vi "Actor Core.vi"(8 "error in":errorcluster, 11 "Hardware Buzzer in":refnum<class "Hardware Buzzer.lvclass">) -> (0 "error out":errorcluster, 3 "Actor out":refnum<class "Actor.lvclass">)   [LabVIEW 2023, in "Hardware Buzzer.lvlib" / "Hardware Buzzer.lvclass"]
doc: "<p>(<strong>Filename</strong>: <span class=\"dnl\">Actor Framework.lvlib:Actor.lvclass:Actor Core.vi</span>)</p>\n<p>Receives messages to the actor, reacts to them, and initiates any error handling that may shut the actor down.</p>\n<p>Descendant classes may override this VI to append parallel tasks for the actor to complete while it handles messages. Overrides use the <a href=\"nihelplauncher://docs/csh?context=lvcore_glang_udclass\">Call Parent Class Method</a> node.</p>"
uses:
  Hardware Buzzer.lvclass
  C:/Program Files/National Instruments/LabVIEW 2024/vi.lib/ActorFramework/Actor/Actor.lvclass
  <vilib>/ActorFramework/Actor/Actor.lvclass
  <vilib>/ActorFramework/Actor/Actor.lvclass/Actor.ctl
  Hardware Buzzer.lvclass/Hardware Buzzer.ctl
  <vilib>/ActorFramework/Message Enqueuer/Message Enqueuer.lvclass/Message Enqueuer.ctl
  Controller/Controller Messages/Set DAQ Panel Reference Msg/Set DAQ Panel Reference Msg.lvclass/Set DAQ Panel Reference Msg.ctl
  Controller/Controller Messages/Buzzer Pressed Msg/Buzzer Pressed Msg.lvclass/Buzzer Pressed Msg.ctl
  <vilib>/DAQmx/read.llb/DAQmx Read (Analog 1D Wfm NChan NSamp).vi
  <vilib>/ActorFramework/Message Enqueuer/Init from Existing Queue.vi
  <vilib>/ActorFramework/Message Enqueuer/Enqueue.vi
  Controller/Controller Messages/Set DAQ Panel Reference Msg/Set DAQ Panel Reference Msg.lvclass
  C:/Program Files/National Instruments/LabVIEW 2024/vi.lib/ActorFramework/Message/Message.lvclass
  Controller/Controller Messages/Buzzer Pressed Msg/Buzzer Pressed Msg.lvclass
  <vilib>/ActorFramework/Stop Msg/Stop Msg.lvclass
  <vilib>/DAQmx/create/channels.llb/DAQmx Create Channel (AI-Voltage-Basic).vi
  <vilib>/DAQmx/configure/timing.llb/DAQmx Timing (Sample Clock).vi
  <vilib>/ActorFramework/Message Priority Queue/Priority Enqueue.vi
  <vilib>/DAQmx/miscellaneous.llb/DAQmx Fill In Error Info.vi
  <vilib>/measure/mamon.llb/Trigger Detection for N Channel.vi
  <vilib>/ActorFramework/Message Enqueuer/Message Enqueuer.lvclass
  <vilib>/measure/NI_MAPro.lvlib
panel:
  out "Waveform Chart":waveform(dbl)[](graph)
  in  "Stop":bool
  in  "3":bool
  in  "2":bool
  in  "1":bool
  in  "0":bool
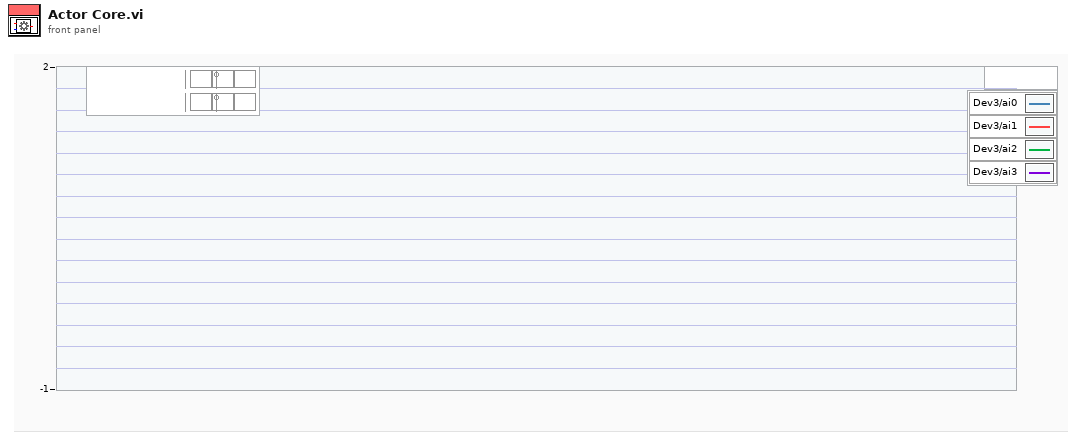
[diagram p1: front panel]
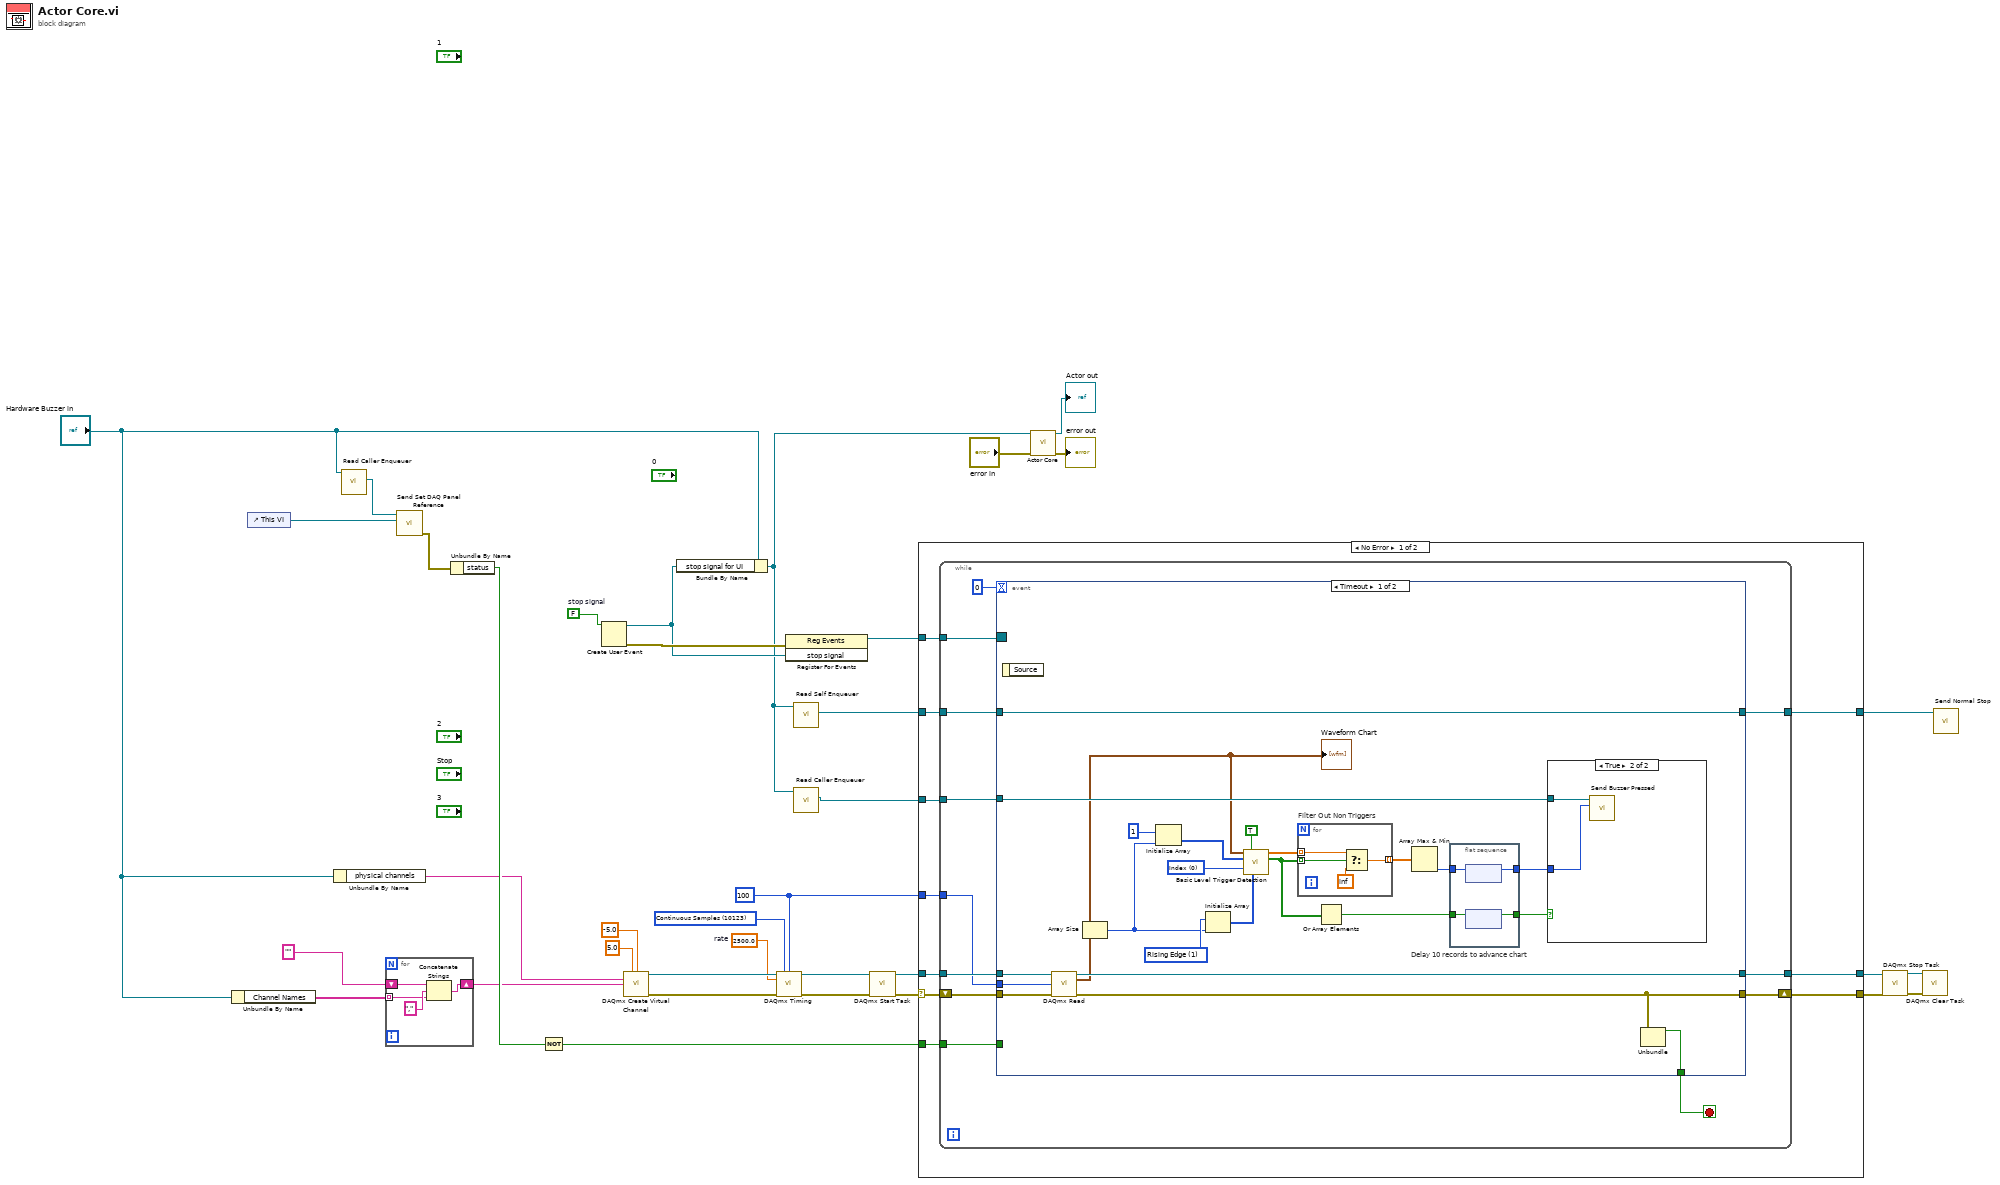
[diagram p0: block diagram]
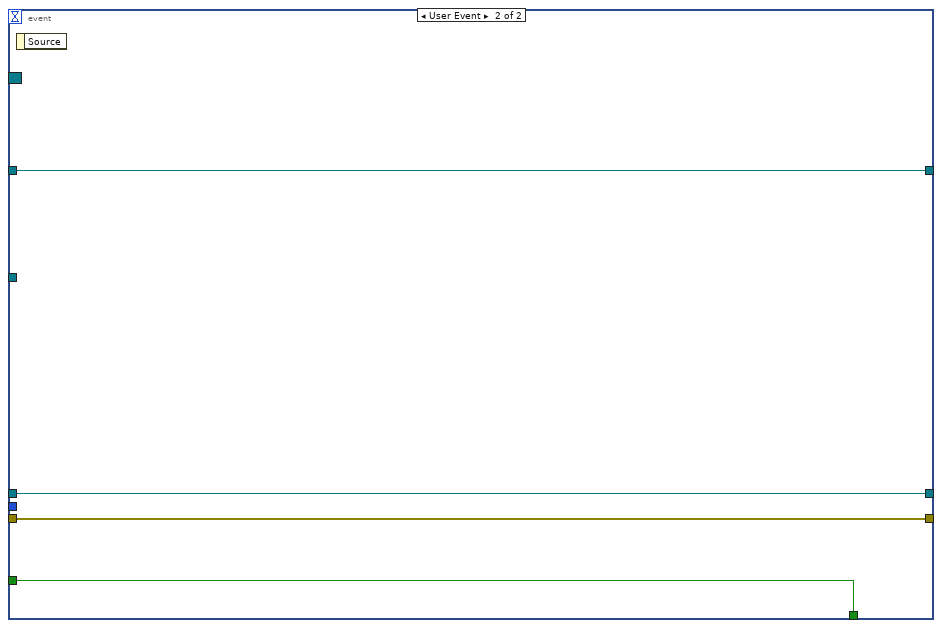
[diagram p3: hidden frame]
diagram:
  w16 = 2500.0  # rate
  w15 = 100 ("samples per channel")
  w17 = 10123 items=["Finite Samples"=10178, "Continuous Samples"=10123, "Hardware Timed Single Point"=12522] ("sample mode")
  w31 = FALSE  # stop signal
  n1 = Unbundle By Name("Hardware Buzzer in") -> ("Channel Names"=w5:string[])
  n2 = control-ref of="This VI"() -> (w29:refnum<vi>)
  n3 = Unbundle By Name("Hardware Buzzer in") -> ("physical channels"=w1:tag)
  n4 = call <vilib>:"Read Caller Enqueuer.vi"("Actor"="Hardware Buzzer in") -> ("Caller Enqueuer"=w30:refnum<class "Message Enqueuer.lvclass">)  [unwired: 10 in]
  n5 = for {
    tunnel: w5 -> [w39] mode=indexing
    shift-right: [w38] -> w4
    shift-left: "" -> [w37]
    n6 = Concatenate Strings(w37, "," ("string"), w39) -> (w38:string)
  }
  n7 = call "Send Set DAQ Panel Reference.vi"("DAQ VI Reference"=w29, "Message Enqueuer"=w30) -> ("error out"=w20:errorcluster)  [unwired: 8 in, 1 out]
  n8 = Unbundle By Name(w20) -> ("status"=w18:bool)
  n9 = Not(x=w18) -> (.not. x?=w19:bool)
  n10 = Create User Event(user event datatype=w31) -> (user event=w32:refnum<user-event>, error out=w33:errorcluster)  [unwired: 1 in]
  n11 = call-poly <vilib>:"DAQmx Create Virtual Channel.vi"("maximum value"=5.0, "minimum value"=-5.0, "physical channels"=w1, "name to assign"=w4) -> ("task out"=w28:refnum<k21>, "error out"=w13:errorcluster)  [unwired: 10 in]
  n12 = Bundle By Name(cluster="Hardware Buzzer in", "stop signal for UI"=w32) -> (w24:refnum<class "Hardware Buzzer.lvclass">)
  n13 = call-poly <vilib>:"DAQmx Timing.vi"("task/channels in"=w28, "sample mode"=w17, "samples per channel"=w15, "rate"=w16, "error in"=w13) -> ("task out"=w11:refnum<k21>, "error out"=w14:errorcluster)  [unwired: 9 in]
  n14 = register-events(error in=w33, w32) -> (reference out=w21:refnum<event-registration>)  [unwired: 1 in, 1 out]
  n15 = call <vilib>:"Read Self Enqueuer.vi"("Actor"=w24) -> ("Self Enqueuer"=w23:refnum<class "Message Enqueuer.lvclass">)  [unwired: 10 in]
  n16 = call <vilib>:"Read Caller Enqueuer.vi"("Actor"=w24) -> ("Caller Enqueuer"=w25:refnum<class "Message Enqueuer.lvclass">)  [unwired: 10 in]
  n17 = call <vilib>:"DAQmx Start Task.vi"("task/channels in"=w11, "error in"=w14) -> ("task out"=w10:refnum<k21>, "error out"=w12:errorcluster)  [unwired: 12 in]
  n18 = case shown="No Error" w12 {
    selector: w12 -> [w44 w100]
    tunnel: w25 -> [w50 _]
    tunnel: w23 -> [w49 w102]
    tunnel: [w48 w102] -> w22
    tunnel: w21 -> [w47 _]
    tunnel: w19 -> [w46 _]
    tunnel: w15 -> [w45 _]
    tunnel: w10 -> [w43 w101]
    tunnel: [w42 w100] -> w9
    tunnel: [w41 w101] -> w8
    frame No Error {
      n19 = while {
        tunnel: w43 -> [w62]
        tunnel: w50 -> [w61]
        tunnel: w49 -> [w59]
        tunnel: [w58] -> w48
        tunnel: w47 -> [w56]
        tunnel: w46 -> [w55]
        tunnel: w45 -> [w54]
        shift-right: [w52] -> w42
        shift-left: w44 -> [w53]
        tunnel: [w51] -> w41
        stop <- w57 stop-if-true
        n20 = event shown="[0] Timeout" {
          selector: w56 -> [_ _]
          dyn-events: _ -> [_ _]
          timeout: 0 -> [_ _]
          tunnel: w62 -> [w85 w96]
          tunnel: w61 -> [w84 _]
          tunnel: w59 -> [w83 w99]
          tunnel: [w83 w99] -> w58
          tunnel: [w65 w98] -> w57
          tunnel: w55 -> [_ w98]
          tunnel: w54 -> [w82 _]
          tunnel: w53 -> [w81 w97]
          tunnel: [w66 w97] -> w52
          tunnel: [w64 w96] -> w51
          event Timeout {
            w76 = u16 1 items=["Falling Edge", "Rising Edge"] ("trigger slope")
            w80 = u16 0 items=["Index", "Time"] ("location mode")
            n21 = event-data() -> ()  [unwired: 1 in, 1 out]
            n22 = call-poly <vilib>:"DAQmx Read.vi"("task/channels in"=w85, "number of samples per channel"=w82, "error in"=w81) -> ("task out"=w64:refnum<k21>, "data"=w63:waveform(dbl)[], "error out"=w66:errorcluster)  [unwired: 10 in]
            "Waveform Chart" <- w63
            n23 = Array Size(array=w63) -> (size(s)=w75:i32)
            n24 = Initialize Array(1 ("samples per channel"), w75) -> (w79:i32[])
            n25 = Initialize Array(w76, w75) -> (w74:u16[])
            n26 = call-poly <vilib>:"Basic Level Trigger Detection.vi"("signal in"=w63, "reset"=TRUE, "level"=w79, "location mode"=w80, "trigger slope"=w74) -> ("trigger locations"=w73:dbl[], "trigger detected?"=w72:bool[])  [unwired: 8 in, 1 out]
            n27 = for "Filter Out Non Triggers" {
              tunnel: w73 -> [w92] mode=indexing
              tunnel: w72 -> [w93] mode=indexing
              tunnel: [w90] -> w70 mode=indexing
              n28 = Select(t=w92, s=w93, f=inf) -> (s? t:f=w90:dbl)
            }
            n29 = Or Array Elements(Boolean array=w72) -> (logical OR=w71:bool)
            n30 = Array Max & Min(array=w70) -> (min index (indices)=w67:i32)  [unwired: 3 out]
            n31 = flat-sequence "Delay 10 records to advance chart" {
              tunnel: w71 -> [w89]
              tunnel: [w88] -> w69
              tunnel: [w87] -> w68
              tunnel: w67 -> [w86]
              frame #0 {
                n32 = feedback #1() -> (w88:i32)  [unwired: 1 in]
                n33 = feedback-in #1(w86) -> ()
                n34 = feedback #2() -> (w87:bool)  [unwired: 1 in]
                n35 = feedback-in #2(w89) -> ()
              }
            }
            n36 = case shown="True" w68 {
              tunnel: w84 -> [_ w95]
              tunnel: w69 -> [_ w94]
              frame False {
              }
              frame True {
                n37 = call "Send Buzzer Pressed.vi"("Buzzer"=w94, "Message Enqueuer"=w95) -> ()  [unwired: 8 in, 2 out]
              }
            }
            n38 = Unbundle(w66) -> ("status"=w65:bool)  [unwired: 2 out]
          }
          event User Event {
            n39 = event-data() -> ()  [unwired: 1 in, 1 out]
          }
        }
      }
    }
    frame Error {
    }
  }
  n40 = call-parent "Actor Core.vi"("error in"="error in", "Actor in"=w24) -> ("error out"=→"error out":errorcluster, "Actor out"=→"Actor out":refnum<class "Actor.lvclass">)  [unwired: 8 in]
  n41 = call <vilib>:"DAQmx Stop Task.vi"("task/channels in"=w8, "error in"=w9) -> ("task out"=w7:refnum<k21>, "error out"=w6:errorcluster)  [unwired: 12 in]
  n42 = call <vilib>:"DAQmx Clear Task.vi"("task in"=w7, "error in"=w6) -> ()  [unwired: 13 in, 1 out]
  n43 = call <vilib>:"Send Normal Stop.vi"("Message Enqueuer"=w22) -> ()  [unwired: 10 in, 1 out]
